vi "nn symbol info.vi"(8 "error in (no error)":errorcluster, 9 "buflen":i32, 10 "buf":T1, 11 "i":i32) -> (0 "error out":errorcluster, 1 "function return":i32, 2 "buf out":T1, 3 "name":string)   [LabVIEW 2013, in "lvnano.lvlib"]
doc: "NN_EXPORT int nn_symbol_info (int i,\n struct nn_symbol_properties *buf, int buflen);"
uses:
  lvnano.lvlib
  <vilib>/Utility/importsl/GetValueByPointer/datatype.ctl
  get last error code.vi
  get error string from code.vi
  <vilib>/Utility/error.llb/Error Cluster From Error Code.vi
  <vilib>/Utility/importsl/GetValueByPointer/GetValueByPointer.xnode
  lvnanomsg.dll
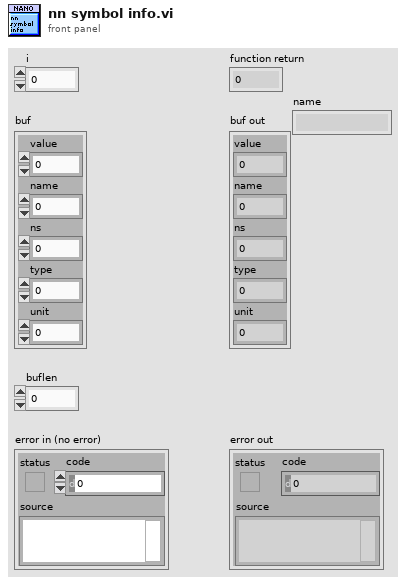
[diagram p1: front panel]
types:
  T1 = cluster{"value":i32, "name":u32, "ns":i32, "type":i32, "unit":i32}
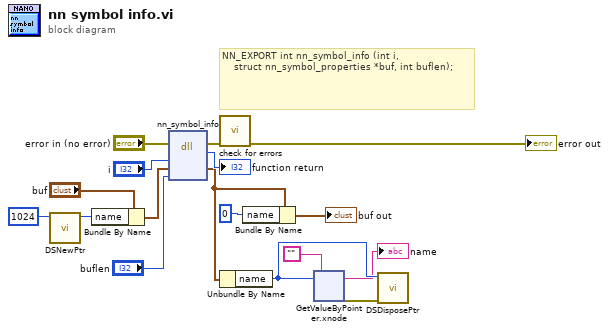
[diagram p0: block diagram]
diagram:
  # "NN_EXPORT int nn_symbol_info (int i,\n    struct nn_symbol_properties *buf, int buflen);"
  n1 = call <vilib>:"DSNewPtr.vi"("Size"=u64 1024) -> ("Pointer"=w13:u64)  [unwired: 9 in, 1 out]
  n2 = Bundle By Name(cluster="buf", "name"=w13) -> (w12:T1)
  n3 = dll-call lib="C:/Users/Daniel/Documents/nanomsg/lvnano/lvnanomsg.*" fn="nn_symbol_info"(error in="error in (no error)", "i"="i", "buf"=w12, "buflen"="buflen") -> (error out=w2:errorcluster, →"function return":i32, "buf"=w7:T1)  [unwired: 4 in, 1 out]
  n4 = call "check for errors.vi"("error in"=w2) -> ("error out"=→"error out":errorcluster)  [unwired: 10 in]
  n5 = Unbundle By Name(w7) -> ("name"=w10:u32)
  n6 = Bundle By Name(cluster=w7, "name"=u32 0) -> (→"buf out":T1)
  n7 = xnode "GetValueByPointer.xnode"("Pointer"=w10, "InputType"="") -> ("Output"=→"name":string, "ErrorOut"=w11:errorcluster)  [unwired: 2 in]
  n8 = call <vilib>:"DSDisposePtr.vi"("error in (no error)"=w11, "Pointer"=w10) -> ()  [unwired: 9 in, 1 out]
